vi "Load DXF.vi"() -> ()   [LabVIEW 2014]
panel:
  out "before substring 2":string
  out "before substring":string
  in  "millisecond multiple":u32
  out "appended array 2":dbl[](array[numeric])
  out "appended array":dbl[](array[numeric])
  out "XY Graph":cluster{dbl[], dbl[]}(graph)
  out "Numeric":i32=30443
  in  "stop":bool
  in  "file (use dialog)":path=path "C:/Users/wwu/Desktop/DXF472/Bald_Eagle.dxf"
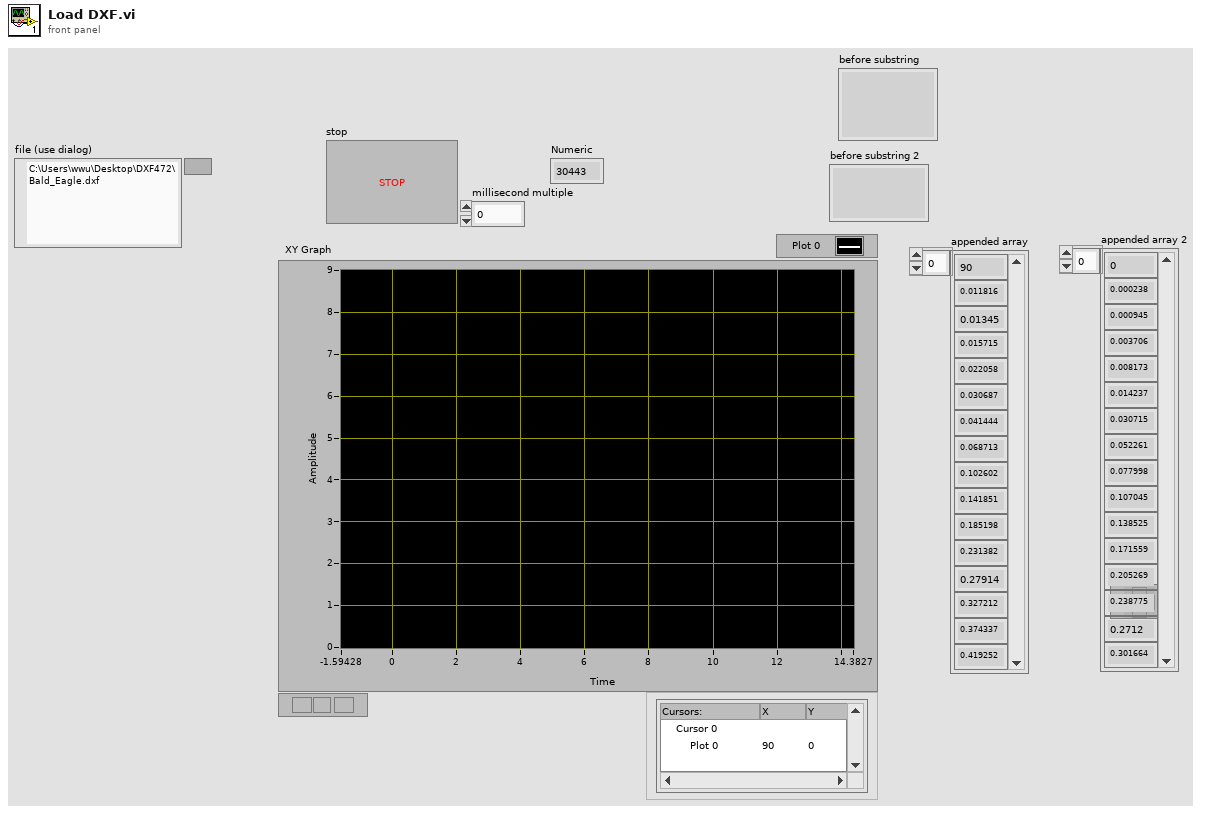
[diagram p1: front panel]
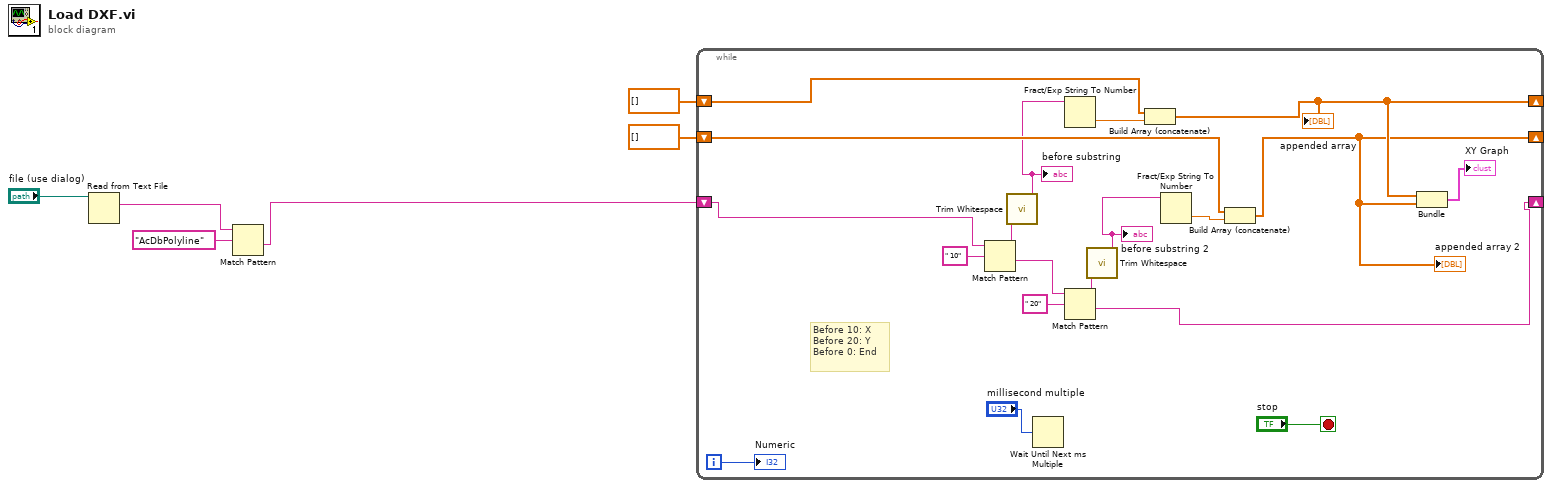
[diagram p0: block diagram]
diagram:
  n1 = Read from Text File(file (use dialog)="file (use dialog)") -> (text=w4:string)  [unwired: 3 in, 3 out]
  n2 = Match Pattern(string=w4, regular expression="AcDbPolyline") -> (after substring=w3:string)  [unwired: 1 in, 3 out]
  n3 = while {
    shift-right: [w8] -> _
    shift-left: w3 -> [w20]
    shift-right: [w13] -> _
    shift-left: dbl[] [] -> [w19]
    shift-right: [w11] -> _
    shift-left: dbl[] [] -> [w16]
    i -> [w14]
    stop <- "stop" stop-if-true
    # "Before 10: X\nBefore 20: Y\nBefore 0: End"
    n4 = Match Pattern(string=w20, regular expression=" 10") -> (before substring=w22:string, after substring=w23:string)  [unwired: 1 in, 2 out]
    n5 = call <vilib>:"Trim Whitespace.vi"("string"=w22) -> ("trimmed string"=w10:string)  [unwired: 1 in]
    "before substring" <- w10
    n6 = Wait Until Next ms Multiple(millisecond multiple="millisecond multiple") -> ()  [unwired: 1 out]
    n7 = Fract/Exp String To Number(string=w10) -> (number=w21:dbl)  [unwired: 3 in, 1 out]
    n8 = Match Pattern(string=w23, regular expression=" 20") -> (before substring=w17:string, after substring=w8:string)  [unwired: 1 in, 2 out]
    n9 = call <vilib>:"Trim Whitespace.vi"("string"=w17) -> ("trimmed string"=w9:string)  [unwired: 1 in]
    "before substring 2" <- w9
    n10 = Build Array (concatenate)(w19, w21) -> (w13:dbl[])
    "appended array" <- w13
    n11 = Fract/Exp String To Number(string=w9) -> (number=w18:dbl)  [unwired: 3 in, 1 out]
    n12 = Build Array (concatenate)(w16, w18) -> (w11:dbl[])
    "appended array 2" <- w11
    n13 = Bundle(w13, w11) -> (→"XY Graph":cluster{dbl[], dbl[]})  [unwired: 1 in]
    "Numeric" <- w14
  }
